vi "runtest add step data to fields.vi"(9 "Step Tag":string, 10 "Step Number":i32, 11 "Fields Array":T1[](array[typedef])) -> (3 "Fields Array":T1[](array[typedef]))   [LabVIEW 2011]
uses:
  server/database/Fields/Field Record.ctl
  server/database/Fields/Field DataTypes.ctl
  server/database/Fields/Field NextItem.ctl
  server/database/Fields/Field System Fields.ctl
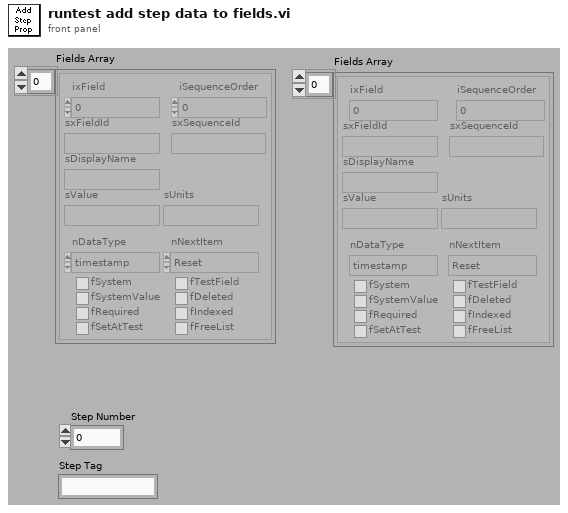
[diagram p1: front panel]
types:
  T1 = typedef "Field Record.ctl" = cluster{"ixField":i32, "iSequenceOrder":i32, "sxFieldId":string, "sxSequenceId":string, "sDisplayName":string, "sValue":string, "sUnits":string, "nDataType":T2, "nNextItem":T3, "fSystem":bool, "fSystemValue":bool, "fRequired":bool, "fSetAtTest":bool, "fTestField":bool, "fDeleted":bool, "fIndexed":bool, "fFreeList":bool}
  T2 = typedef "Field DataTypes.ctl" = enum32{"text", "numeric", "list", "timestamp", "boolean"}
  T3 = typedef "Field NextItem.ctl" = enum32{"Reset", "Retain", "Auto-Increment"}
  T4 = typedef "Field System Fields.ctl" = enum32{"Company", "End_Timestamp", "Model_Number", "Operator", "Serial_Number", "Start_Timestamp", "Step_Number", "Step_Tag", "Test_Run", "Test_Sequence", "Test_Station", "Test_Station_Name", "Test_Status", "Test_Type", "Test_Version", "Spartan_Version_Created", "Spartan_Version_Current"}
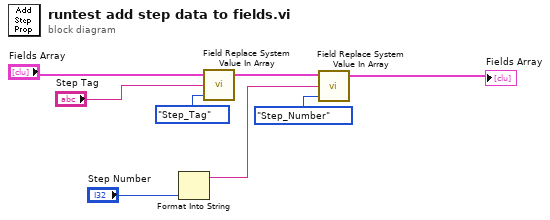
[diagram p0: block diagram]
diagram:
  n1 = Format Into String("Step Number") -> (resulting string=w1:string)  [unwired: 3 in, 1 out]
  n2 = call "Field Replace System Value In Array.vi"("System Field to Replace (Serial Number)"=Field_System_Fields."Step_Tag", "Field Value Replacement Data (\"\")"="Step Tag", "Fields Array In"="Fields Array") -> ("Fields Array Out"=w5:T1[])  [unwired: 1 in, 1 out]
  n3 = call "Field Replace System Value In Array.vi"("System Field to Replace (Serial Number)"=Field_System_Fields."Step_Number", "Field Value Replacement Data (\"\")"=w1, "Fields Array In"=w5) -> ("Fields Array Out"=→"Fields Array":T1[])  [unwired: 1 in, 1 out]
